vi "addCheckIN.vi"(0 "reference in":refnum<class "Project Panels.lvclass">=refnum, 11 "error in (no error)":errorcluster) -> (4 "reference out":refnum<class "Project Panels.lvclass">, 8 "saved?":bool, 15 "error out":errorcluster={"status"=TRUE, "code"=1556, "source"="In Place Element Structure in Project Panels.lvclass:addCheckIN.vi"})   [LabVIEW 2015, in "Project Panels.lvclass"]
uses:
  Project Panels.lvclass
  <vilib>/Utility/miscctls.llb/LVRowAndColumnTypeDef.ctl
  deviceState.ctl
  SYS/Items Controller_llb/Items Controller.lvclass
  APP/checkIN_class/checkIN.lvclass
panel:
  out "Cell Position":T1={"Row"=0, "Column"=4}
  out "title":string="Add Check IN"
  in  "getPDFFile":bool
  in  "updateData":bool
  in  "Quantity":i32
  in  "Description:":string
  in  "S/N:":string caption="Add more than one seprated by a \",\" without space"
  in  "P/N:":string
  out "dataIN":string[][](table)
  in  "Invoice Date:":string caption="(dd/mm/yyyy)"
  in  "Invoice Type:":string
  in  "Invoice Number:":string
  in  "ADD":bool
  in  "Date IN:":string caption="(dd/mm/yyyy)"
  out "Status bar":string="Fill in all and press the DONE button....."
  in  "Stop Button":bool
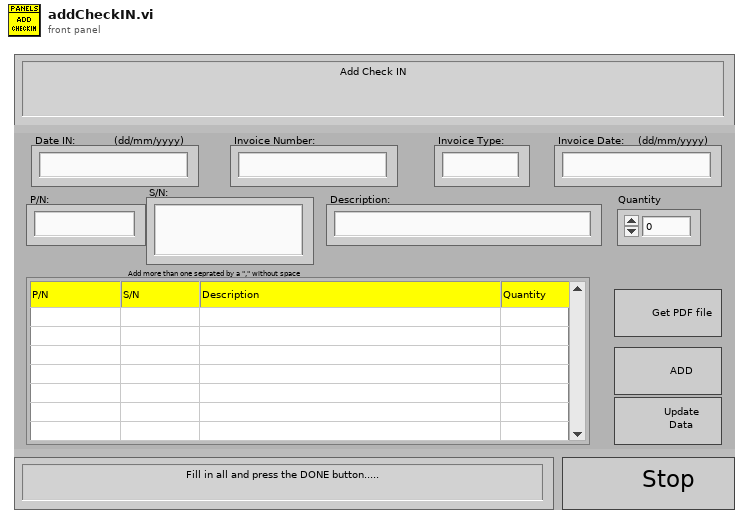
[diagram p1: front panel]
types:
  T1 = typedef "LVRowAndColumnTypeDef.ctl" = cluster{"Row":i32, "Column":i32}
  T2 = cluster{"P/N":string, "S/N":string, "Description":string, "Quantity":i32}
  T3 = typedef "Project Panels.lvclass/deviceState.ctl" = enum16{"check", "initiate", "waitEvent", "dataFromPDF", "getDetails", "TSR", "save", "close", "stop"}
  T4 = typedef "Project Panels.lvclass/ObjectAttributesRef.ctl" = refnum<data-value>
  T5 = typedef "Project Panels.lvclass/ObjectAttributes.ctl" = cluster{"MyAttribute":dbl, "device_controller_ref":refnum<class "Devices Controller.lvclass">, "file_controller_ref":refnum<class "File Controller.lvclass">, "item_controller_ref":refnum<class "Items Controller.lvclass">, "item_tables":cluster{"checkIN":string[][], "checkOUT":string[][], "storage":string[][]}, "quickbook_table":cluster{"notes":string[][]}, "notification_controller_ref":refnum<class "Notification Controller.lvclass">, "partstracking_controller_ref":refnum<class "PartsTracking Controller.lvclass">, "product_tables":cluster{"k4b2":string[][], "fitmate":string[][], "RMR":string[][], "CPET":string[][], "BP":string[][], "PP":string[][], "k5":string[][], "bb-pft":string[][]}, "rowsColour":u32[], "low_resolution?":bool}
  T6 = typedef "LVPoint32TypeDef.ctl" = cluster{"Horizontal":i32, "Vertical":i32}
  T7 = cluster{"checkIN_ref":refnum<class "checkIN.lvclass">, "checkOUT_ref":refnum<class "checkOUT.lvclass">, "item_ref":refnum<class "item.lvclass">}
  T8 = cluster{"numItems":string, "date":string, "numInvoice":string, "P/N":string[], "S/N":string[], "Descr":string[], "Qty":string[]}
  T9 = enum16{"Left Button", "Center Button", "Right Button", "Window Close"}
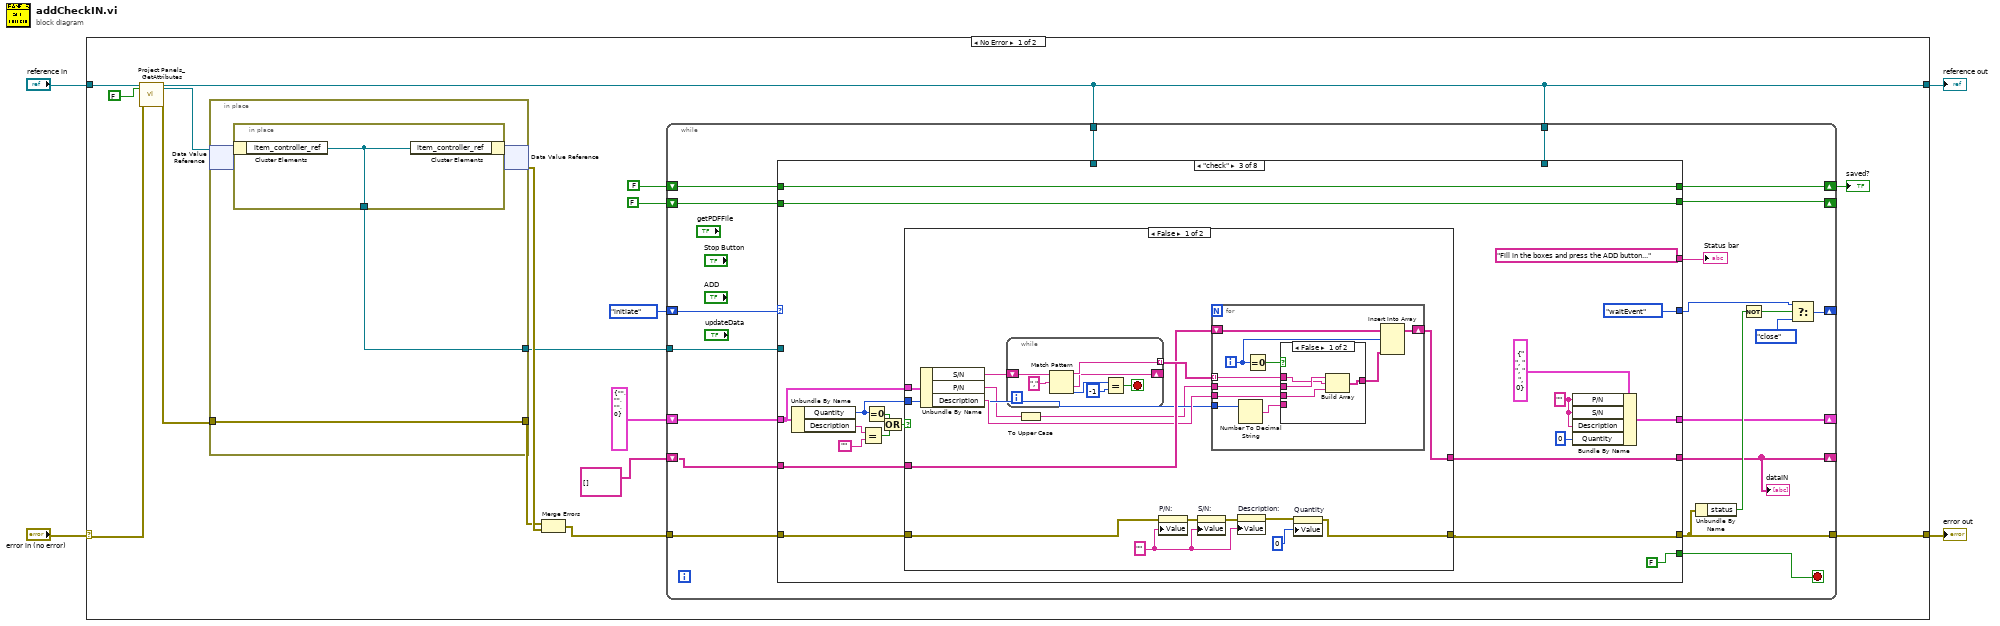
[diagram p0: block diagram]
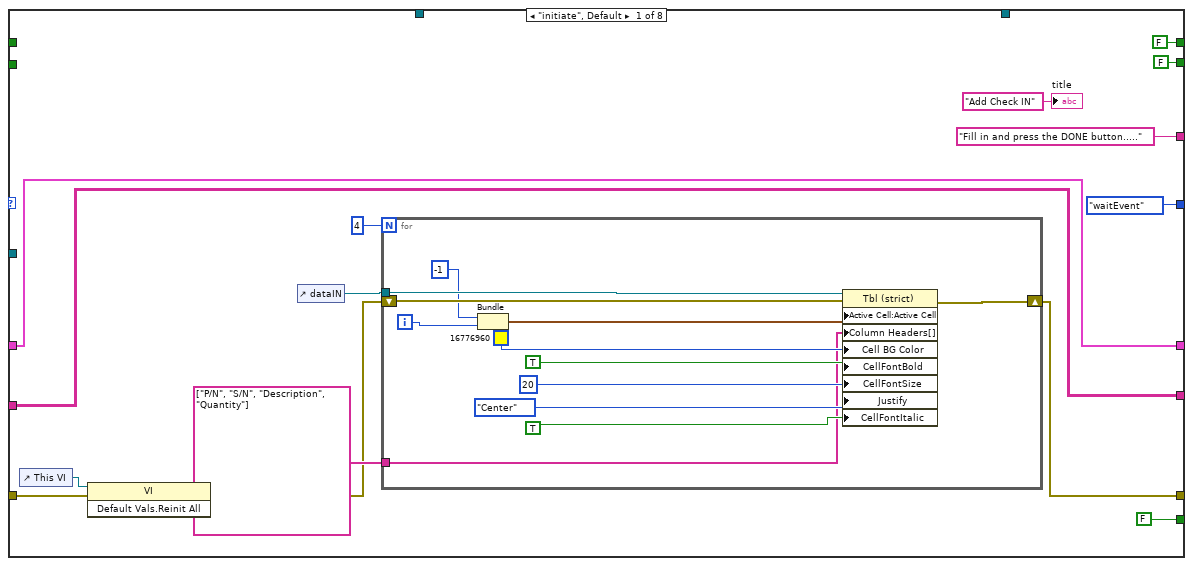
[diagram p2: hidden frame]
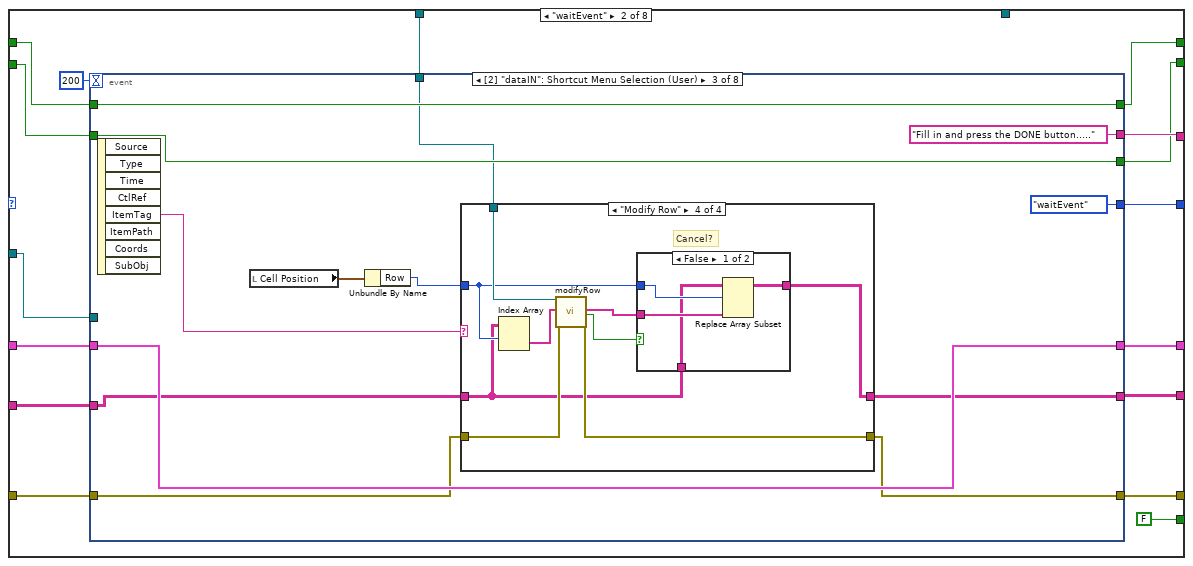
[diagram p3: hidden frame]
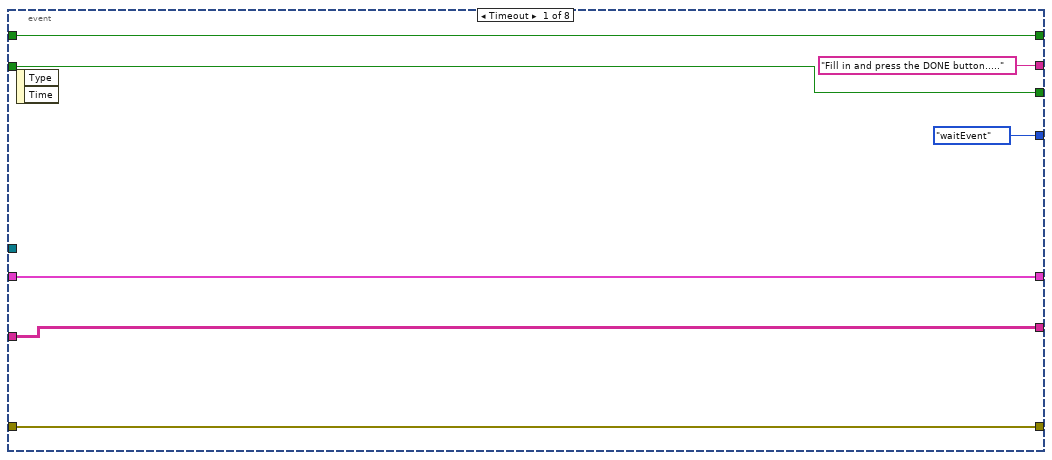
[diagram p4: hidden frame]
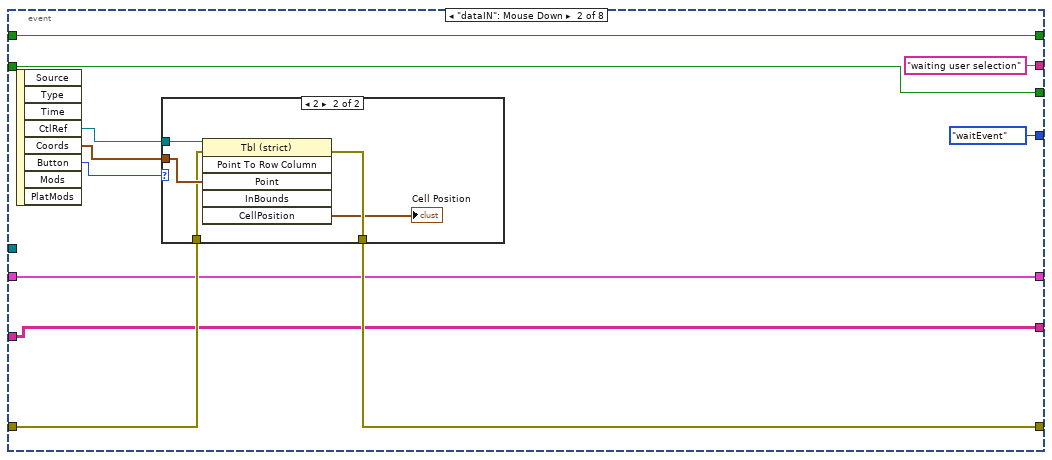
[diagram p5: hidden frame]
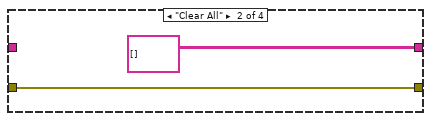
[diagram p8: hidden frame]
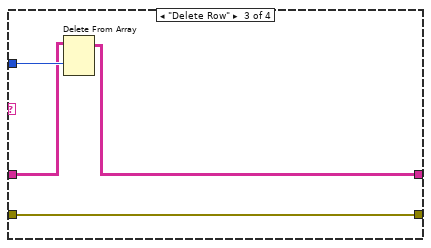
[diagram p9: hidden frame]
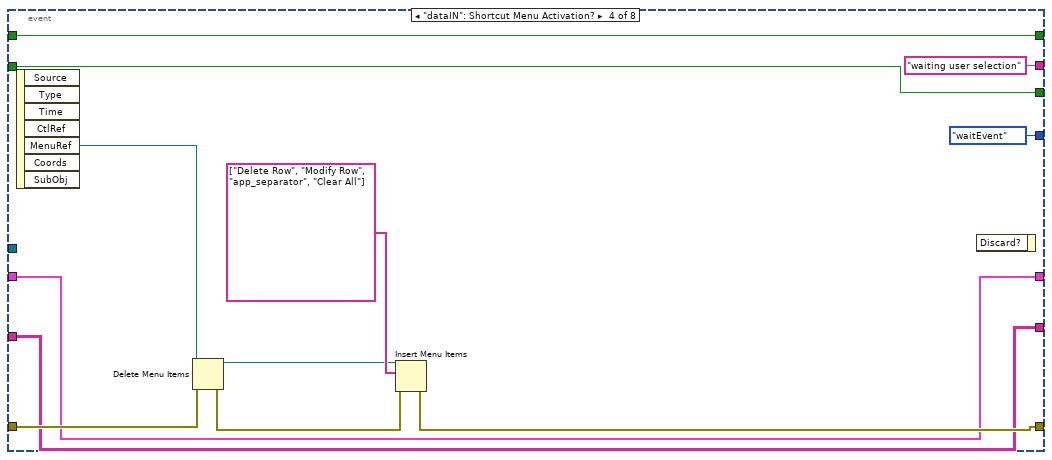
[diagram p11: hidden frame]
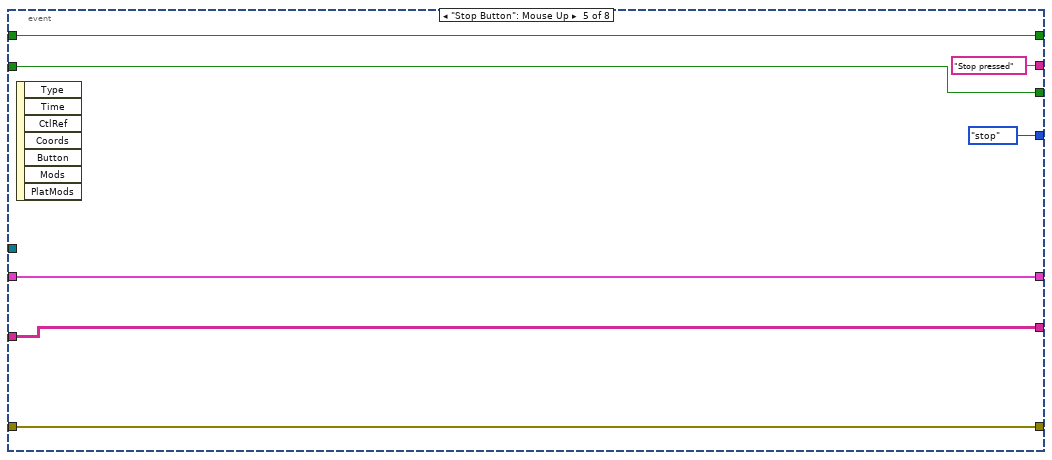
[diagram p12: hidden frame]
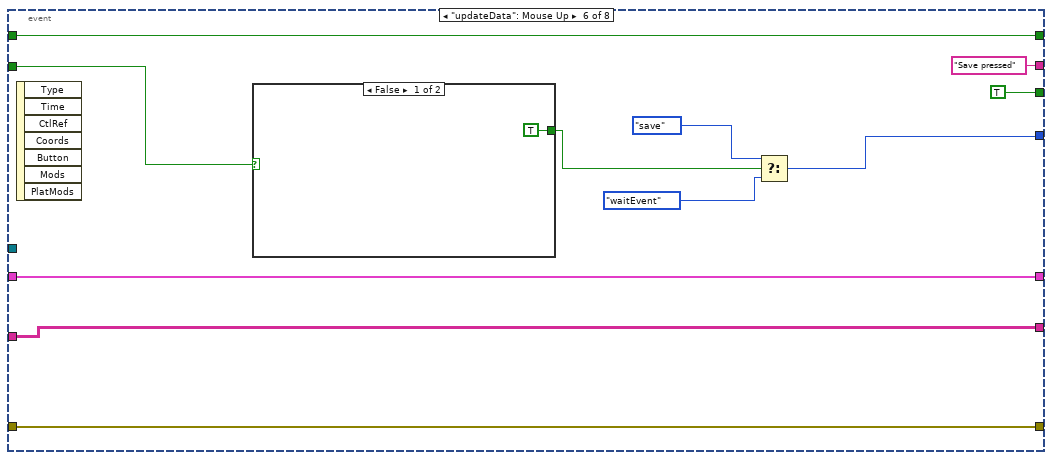
[diagram p13: hidden frame]
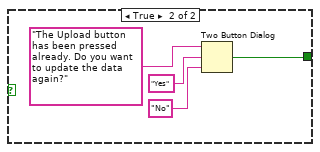
[diagram p14: hidden frame]
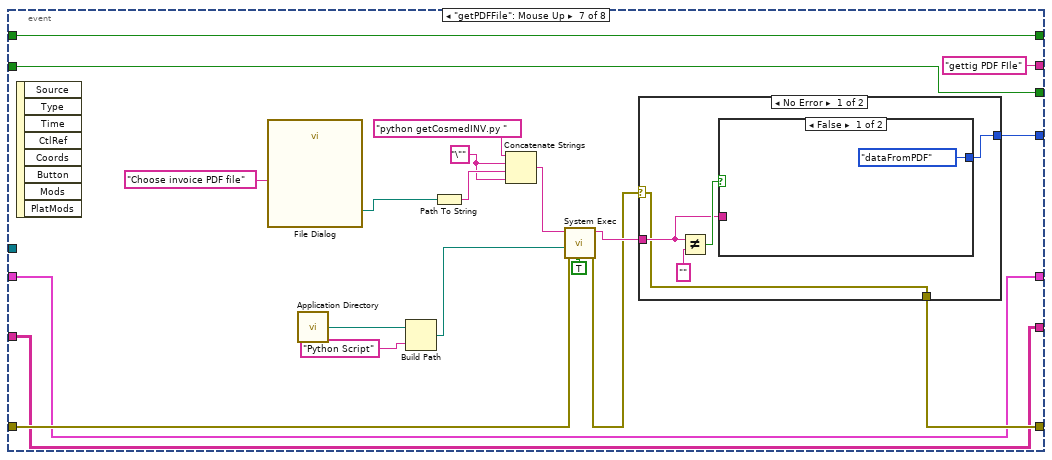
[diagram p15: hidden frame]
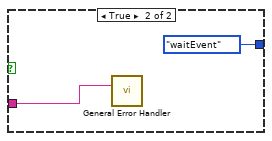
[diagram p16: hidden frame]
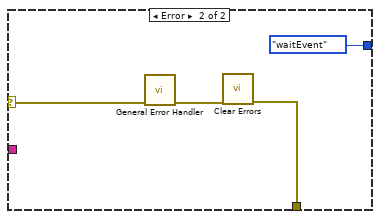
[diagram p17: hidden frame]
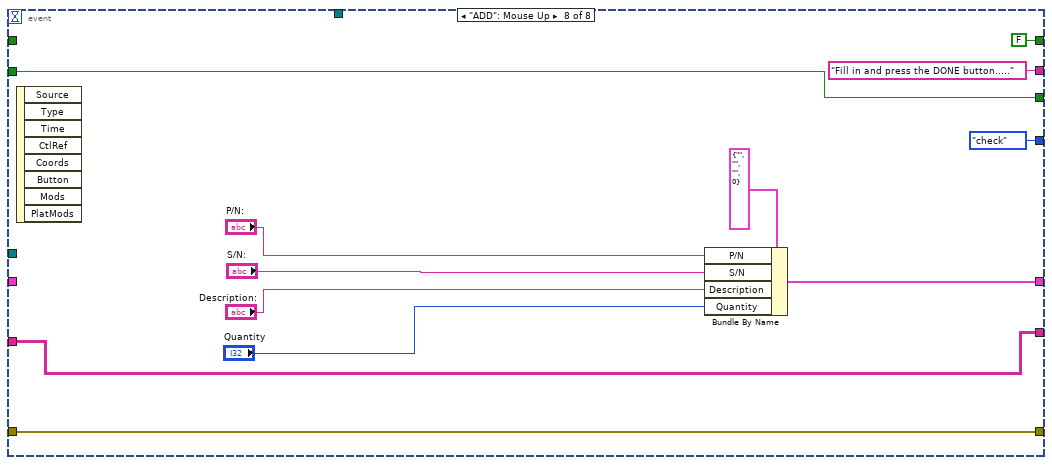
[diagram p18: hidden frame]
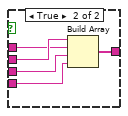
[diagram p19: hidden frame]
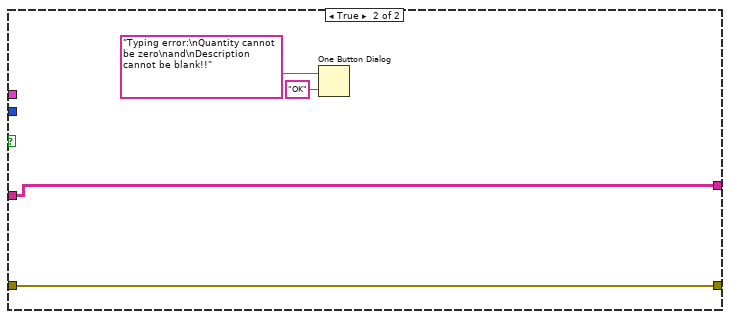
[diagram p20: hidden frame]
diagram:
  n1 = case shown="No Error" "error in (no error)" {
    selector: "error in (no error)" -> [w17 w422]
    tunnel: [w14 w422] -> w3
    tunnel: [w5 w421] -> w1
    tunnel: "reference in" -> [w19 w421]
    frame No Error {
      n2 = call "Project Panels_GetAttributes.vi"("reference in"=w19, "return data? (T)"=FALSE, "error in (no error)"=w17) -> ("reference out"=w5:refnum<class "Project Panels.lvclass">, "attributes ref"=w15:T4, "error out"=w16:errorcluster)  [unwired: 13 in, 1 out]
      n3 = in-place {
        in-place-border: w16 -> [w417]
        in-place-border: [w417] -> w20
        in-place-border: [w416] -> w11
        n4 = in-place-dvr #1(w15) -> (w418:T5)  [unwired: 1 out]
        n5 = in-place {
          in-place-border: [w420] -> w416
          n6 = in-place-cluster #2(w418) -> ("item_controller_ref"=w420:refnum<class "Items Controller.lvclass">)
          n7 = in-place-cluster #2("item_controller_ref"=w420) -> (w419:T5)
        }
        n8 = in-place-dvr #1(w419) -> (w21:errorcluster)  [unwired: 1 out]
      }
      n9 = Merge Errors(w20, w21) -> (w12:errorcluster)
      n10 = while {
        tunnel: w12 -> [w42]
        tunnel: [w24] -> w14
        shift-right: [w39] -> _
        shift-left: deviceState."initiate" ("state") -> [w41]
        tunnel: w5 -> [w35]
        tunnel: w11 -> [w33]
        shift-right: [w31] -> _
        shift-left: T2 {"P/N"="", "S/N"="", "Description"="", "Quantity"=0} -> [w30]
        shift-right: [w23] -> _
        shift-left: string[][] [] ("dataIN 2") -> [w29]
        shift-right: [w27] -> w7
        shift-left: FALSE -> [w28]
        shift-right: [w25] -> _
        shift-left: FALSE -> [w26]
        tunnel: w5 -> [w22]
        stop <- w34 stop-if-true
        n11 = case shown="\"check\"" w41 {
          tunnel: w42 -> [w53 w85 w240 w310 w335 w350 w381 w395]
          tunnel: [w48 w84 w231 w308 w335 w344 w381 w395] -> w24
          tunnel: [deviceState."waitEvent" ("state") w82 deviceState."waitEvent" ("f") deviceState."waitEvent" ("f") deviceState."stop" ("f") deviceState."waitEvent" ("f") deviceState."close" ("f") w391] -> w40
          tunnel: w35 -> [_ _ _ _ _ _ _ _]
          tunnel: [FALSE FALSE FALSE FALSE FALSE FALSE TRUE FALSE] -> w34
          tunnel: w33 -> [_ w73 _ w307 _ w351 _ _]
          tunnel: ["Fill in and press the DONE button....." ("Status bar") w80 "Fill in the boxes and press the ADD button..." ("Status bar") "Check data imported from PDF" ("Status bar") "" ("Status bar") "Wait while the new data are saved in the inventory" ("Status bar") "" ("Status bar") w392] -> w32
          tunnel: [w46 w79 w234 w306 w332 w356 w384 w394] -> w31
          tunnel: w30 -> [w46 w78 w236 w306 w332 w356 w384 w394]
          tunnel: w29 -> [w45 w77 w239 w299 w331 w341 w383 w393]
          tunnel: [w45 w76 w238 w298 w331 w341 w383 w393] -> w23
          tunnel: w28 -> [_ w75 w230 _ w330 _ w382 w390]
          tunnel: [FALSE w74 w230 FALSE w330 TRUE w382 w390] -> w27
          tunnel: w26 -> [_ w71 w224 w290 w329 w337 w380 w389]
          tunnel: [FALSE w72 w224 w290 w329 w337 w380 w389] -> w25
          tunnel: w22 -> [_ w70 _ _ _ _ _ _]
          frame "initiate", Default {
            n12 = control-ref of="This VI"() -> (w54:refnum<vi>)
            n13 = invoke class="VI" method="Default Vals.Reinit All"(reference=w54, error in=w53) -> (error out=w49:errorcluster)  [unwired: 1 in, 2 out]
            n14 = control-ref of="dataIN"() -> (w50:refnum<vi>)
            n15 = for {
              N: 4 -> [_]
              tunnel: w50 -> [w67]
              shift-right: [w68] -> w48
              shift-left: w49 -> [w69]
              tunnel: string[] ["P/N", "S/N", "Description", "Quantity"] ("Column Header Strings[]") -> [w58]
              i -> [w65]
              n16 = Bundle("index"=-1, w65) -> (w66:cluster{"index":i32, i32})  [unwired: 1 in]
              n17 = property on="Property Node" class="Tbl (strict)"(reference=w67, error in=w69, "Active Cell:Active Cell"=w66, "Column Headers[]"=w58, "Cell BG Color"=u32 16776960, "CellFontBold"=TRUE ("Active Cell:Cell Font:Bold"), "CellFontSize"=u32 20 ("Active Cell:Cell Font:Size"), "Justify"=enum16{"Left", "Center", "Right"}."Center" ("Active Cell:Cell Justification"), "CellFontItalic"=TRUE ("Active Cell:Cell Font:Italic")) -> (error out=w68:errorcluster)  [unwired: 1 out]
            }
            "title" <- "Add Check IN" ("title")
          }
          frame "waitEvent" {
            n18 = event shown="[2] \"dataIN\": Shortcut Menu Selection (User)" {
              selector: _ -> [_ _ _ _ _ _ _ _]
              dyn-events: _ -> [_ _ _ _ _ _ _ _]
              timeout: 200 -> [_ _ _ _ _ _ _ _]
              tunnel: w85 -> [w92 w103 w112 w154 w162 w174 w196 w223]
              tunnel: [w92 w102 w111 w152 w162 w174 w183 w223] -> w84
              tunnel: [deviceState."waitEvent" ("f") deviceState."waitEvent" ("f") deviceState."waitEvent" ("f") deviceState."waitEvent" ("f") deviceState."stop" ("f") w165 w186 deviceState."check" ("f")] -> w82
              tunnel: ["Fill in and press the DONE button....." ("Status bar") "waiting user selection" ("Status bar") "Fill in and press the DONE button....." ("Status bar") "waiting user selection" ("Status bar") "Stop pressed" ("Status bar") "Save pressed" ("Status bar") "gettig PDF FIle" ("Status bar") "Fill in and press the DONE button....." ("Status bar")] -> w80
              tunnel: [w89 w96 w122 w149 w160 w172 w181 w217] -> w79
              tunnel: w78 -> [w89 w96 w122 w149 w160 w172 w181 _]
              tunnel: w77 -> [w86 w97 w116 w150 w159 w171 w182 w214]
              tunnel: [w86 w97 w115 w150 w159 w171 w182 w214] -> w76
              tunnel: w75 -> [w88 w94 w119 w145 w158 w170 w198 _]
              tunnel: [w88 w94 w119 w145 w158 w170 w198 FALSE] -> w74
              tunnel: w73 -> [_ _ _ _ _ _ _ _]
              tunnel: [w87 w95 w120 w146 w157 TRUE w180 w212] -> w72
              tunnel: w71 -> [w87 w95 w120 w146 w157 w168 w180 w212]
              tunnel: w70 -> [_ _ w110 _ _ _ _ _]
              event Timeout {
                n19 = event-data() -> ()  [unwired: 1 in, 2 out]
              }
              event "dataIN": Mouse Down {
                n20 = event-data() -> ("CtlRef"=w99:refnum<vi>, "Coords"=w100:T6, "Button"=w101:u16)  [unwired: 1 in, 5 out]
                n21 = case shown="2" w101 {
                  tunnel: w99 -> [_ w109]
                  tunnel: w100 -> [_ w108]
                  tunnel: w103 -> [w104 w107]
                  tunnel: [w104 w106] -> w102
                  frame 0, Default {
                  }
                  frame 2 {
                    n22 = invoke class="Tbl (strict)" method="Point To Row Column"(reference=w109, error in=w107, "Point"=w108) -> (error out=w106:errorcluster, "CellPosition"=→"Cell Position":T1)  [unwired: 3 in, 4 out]
                  }
                }
              }
              event "dataIN": Shortcut Menu Selection (User) {
                n23 = event-data() -> ("ItemTag"=w114:string)  [unwired: 1 in, 7 out]
                n24 = local read "Cell Position"() -> (w117:T1)
                n25 = Unbundle By Name(w117) -> ("Row"=w113:i32)
                n26 = case shown="\"Modify Row\"" w114 {
                  tunnel: w116 -> [w124 _ w129 w133]
                  tunnel: [w124 string[][] [] ("dataIN 2") w128 w137] -> w115
                  tunnel: w113 -> [_ _ w130 w134]
                  tunnel: w112 -> [w123 w125 w127 w139]
                  tunnel: [w123 w125 w127 w138] -> w111
                  tunnel: w110 -> [_ _ _ w135]
                  frame "False", Default {
                  }
                  frame "Clear All" {
                  }
                  frame "Delete Row" {
                    n27 = Delete From Array(array=w129, index (row)=w130) -> (array with subset deleted=w128:string[][])  [unwired: 2 in, 1 out]
                  }
                  frame "Modify Row" {
                    # "Cancel?"
                    n28 = Index Array(array=w133, index (row)=w134) -> (element=w132:string[])  [unwired: 1 in]
                    n29 = call-dynamic "modifyRow.vi"("reference in"=w135, "Row In"=w132, "error in (no error)"=w139) -> ("Row"=w136:string[], "Cancel?"=w131:bool, "error out"=w138:errorcluster)  [unwired: 13 in, 1 out]
                    n30 = case shown="False" w131 {
                      tunnel: [w143 w144] -> w137
                      tunnel: w136 -> [w142 _]
                      tunnel: w134 -> [w141 _]
                      tunnel: w133 -> [w140 w144]
                      frame False {
                        n31 = Replace Array Subset(array=w140, new element=w142, index (row)=w141) -> (w143:string[][])  [unwired: 1 in]
                      }
                      frame True {
                      }
                    }
                  }
                }
              }
              event "dataIN": Shortcut Menu Activation? {
                n32 = event-data() -> ("MenuRef"=w151:refnum<k9>)  [unwired: 1 in, 6 out]
                n33 = Delete Menu Items(6:w154, 9:w151) -> (0:w153:errorcluster, 3:w155:refnum<k9>)  [unwired: 2 in]
                n34 = Insert Menu Items(6:w153, 8:string[] ["Delete Row", "Modify Row", "app_separator", "Clear All"] ("item names"), 9:w155) -> (0:w152:errorcluster)  [unwired: 3 in, 2 out]
                n35 = event-data() -> ()  [unwired: 2 in, 1 out]
              }
              event "Stop Button": Mouse Up {
                n36 = event-data() -> ()  [unwired: 1 in, 7 out]
              }
              event "updateData": Mouse Up {
                n37 = event-data() -> ()  [unwired: 1 in, 7 out]
                n38 = case shown="False" w168 {
                  tunnel: [TRUE ("T button?") w176] -> w167
                  frame False {
                  }
                  frame True {
                    n39 = Two Button Dialog(message="The Upload button has been pressed already. Do you want to update the data again?", 1:"No" ("F button name (\"Cancel\")"), 2:"Yes" ("T button name (\"OK\")")) -> (T button?=w176:bool)
                  }
                }
                n40 = Select(t=deviceState."save" ("f"), s=w167, f=deviceState."waitEvent") -> (s? t:f=w165:T3)
              }
              event "getPDFFile": Mouse Up {
                w191 = "\"" ("string")
                n41 = event-data() -> ()  [unwired: 1 in, 8 out]
                n42 = call "File Dialog"("prompt"="Choose invoice PDF file") -> ("selected path"=w195:path)  [unwired: 11 in, 3 out]
                n43 = call <vilib>:"Application Directory.vi"() -> ("Application Directory"=w189:path)
                n44 = Build Path(base path=w189, name or relative path="Python Script" ("string")) -> (appended path=w187:path)
                n45 = Path To String(path=w195) -> (string=w192:string)
                n46 = Concatenate Strings("python getCosmedINV.py " ("command line"), w191, w192, w191) -> (w190:string)
                n47 = call <vilib>:"System Exec.vi"("run minimized? (F)"=TRUE, "error in (no error)"=w196, "working directory"=w187, "command line"=w190) -> ("error out"=w184:errorcluster, "standard output"=w185:string)  [unwired: 2 in, 4 out]
                n48 = case shown="No Error" w184 {
                  selector: w184 -> [w200 w210]
                  tunnel: [w202 deviceState."waitEvent" ("f")] -> w186
                  tunnel: w185 -> [w201 _]
                  tunnel: [w200 w208] -> w183
                  frame No Error {
                    n49 = Not Equal?(x=w201, y="") -> (x != y?=w203:bool)
                    n50 = case shown="False" w203 {
                      tunnel: w201 -> [_ w206]
                      tunnel: [deviceState."dataFromPDF" ("f") deviceState."waitEvent" ("f")] -> w202
                      frame False {
                      }
                      frame True {
                        n51 = call <vilib>:"General Error Handler.vi"("[error source] (\" \")"=w206) -> ()  [unwired: 10 in, 5 out]
                      }
                    }
                  }
                  frame Error {
                    n52 = call <vilib>:"General Error Handler.vi"("error in (no error)"=w210) -> ("error out"=w209:errorcluster)  [unwired: 10 in, 4 out]
                    n53 = call <vilib>:"Clear Errors.vi"("error in (no error)"=w209) -> ("error out"=w208:errorcluster)  [unwired: 5 in, 1 out]
                  }
                }
              }
              event "ADD": Mouse Up {
                n54 = event-data() -> ()  [unwired: 1 in, 8 out]
                n55 = Bundle By Name(cluster=T2 {"P/N"="", "S/N"="", "Description"="", "Quantity"=0}, "P/N"="P/N:", "S/N"="S/N:", "Description"="Description:", "Quantity"="Quantity") -> (w217:T2)
              }
            }
          }
          frame "check" {
            w233 = "" ("P/N")
            n56 = Unbundle By Name(w236) -> ("Quantity"=w237:i32, "Description"=w229:string)
            n57 = Equal?(x=w229, y="") -> (x = y?=w226:bool)
            n58 = Equal To 0?(x=w237) -> (x = 0?=w225:bool)
            n59 = Or(x=w225, y=w226) -> (x .or. y?=w227:bool)
            n60 = case shown="False" w227 {
              tunnel: w240 -> [w247 w289]
              tunnel: [w246 w289] -> w231
              tunnel: w239 -> [w257 w286]
              tunnel: [w253 w286] -> w238
              tunnel: w237 -> [w254 _]
              tunnel: w236 -> [w259 _]
              frame False {
                w251 = "" ("P/N:")
                n61 = Unbundle By Name(w259) -> ("S/N"=w256:string, "P/N"=w245:string, "Description"=w255:string)
                n62 = while {
                  tunnel: [w284] -> w258 mode=indexing
                  shift-right: [w280] -> _
                  shift-left: w256 -> [w279]
                  stop <- w283 stop-if-true
                  n63 = Match Pattern(string=w279, regular expression=",") -> (before substring=w284:string, after substring=w280:string, offset past match=w282:i32)  [unwired: 1 in, 1 out]
                  n64 = Equal?(x=w282, y=-1) -> (x = y?=w283:bool)
                }
                n65 = To Upper Case(1:w245) -> (0:w244:string)
                n66 = property on="P/N:" class="Str"(error in=w247, "Value"=w251) -> (error out=w248:errorcluster)  [unwired: 1 in, 1 out]
                n67 = property on="S/N:" class="Str"(error in=w248, "Value"=w251) -> (error out=w249:errorcluster)  [unwired: 1 in, 1 out]
                n68 = for {
                  tunnel: w258 -> [w268] mode=indexing
                  tunnel: w244 -> [w269]
                  tunnel: w255 -> [w267]
                  shift-right: [w265] -> w253
                  shift-left: w257 -> [w266]
                  tunnel: w254 -> [w263]
                  i -> [w260]
                  n69 = Number To Decimal String(number=w263) -> (decimal integer string=w262:string)  [unwired: 1 in]
                  n70 = Equal To 0?(x=w260) -> (x = 0?=w261:bool)
                  n71 = case shown="False" w261 {
                    tunnel: w269 -> [w271 w278]
                    tunnel: w268 -> [w270 w277]
                    tunnel: w267 -> [w272 w276]
                    tunnel: [w273 w275] -> w264
                    tunnel: w262 -> [_ w274]
                    frame False {
                      n72 = Build Array(w271, w270, w272) -> (w273:string[])
                    }
                    frame True {
                      n73 = Build Array(w278, w277, w276, w274) -> (w275:string[])
                    }
                  }
                  n74 = Insert Into Array(array=w266, index (row)=w260, new element=w264) -> (w265:string[][])  [unwired: 1 in]
                }
                n75 = property on="Description:" class="Str"(error in=w249, "Value"=w251) -> (error out=w250:errorcluster)  [unwired: 1 in, 1 out]
                n76 = property on="Quantity" class="DigNum (strict)"(error in=w250, "Value"=0 ("Quantity")) -> (error out=w246:errorcluster)  [unwired: 1 in, 1 out]
              }
              frame True {
                n77 = One Button Dialog(message="Typing error:\nQuantity cannot be zero\nand\nDescription cannot be blank!!", button name ("OK")="OK") -> ()  [unwired: 1 out]
              }
            }
            n78 = Bundle By Name(cluster=T2 {"P/N"=" ", "S/N"=" ", "Description"=" ", "Quantity"=0}, "P/N"=w233, "S/N"=w233, "Description"=w233, "Quantity"=0) -> (w234:T2)
          }
          frame "dataFromPDF" {
            n79 = call "getItemsRefs.vi"("error in (no error)"=w310, "reference in"=w307) -> ("error out"=w309:errorcluster, "itemsRef"=w312:T7)  [unwired: 7 in, 1 out]
            n80 = call <vilib>:"Application Directory.vi"() -> ("Application Directory"=w305:path)
            n81 = Unbundle By Name(w312) -> ("checkIN_ref"=w311:refnum<class "checkIN.lvclass">)
            n82 = Get Date/Time In Seconds() -> (seconds since 1Jan1904=w291:timestamp)
            n83 = Build Path(base path=w305, name or relative path="Python Script\\results.txt" ("string")) -> (appended path=w303:path)
            n84 = Get Date/Time String(seconds (now)=w291) -> (date string=w292:string)  [unwired: 2 in, 1 out]
            n85 = call "getPDFData.vi"("reference in"=w311, "file (use dialog)"=w303, "error in (no error)"=w309) -> ("dataOUT"=w302:T8, "error out"=w308:errorcluster)  [unwired: 14 in, 1 out]
            n86 = Unbundle By Name(w302) -> ("date"=w300:string, "numInvoice"=w301:string, "P/N"=w297:string[], "S/N"=w296:string[], "Descr"=w295:string[], "Qty"=w294:string[])
            n87 = local write "Invoice Type:"("REM" ("Invoice Type:")) -> ()
            n88 = local write "Date IN:"(w292) -> ()
            n89 = local write "Invoice Number:"(w301) -> ()
            n90 = local write "Invoice Date:"(w300) -> ()
            n91 = for {
              tunnel: w297 -> [w323] mode=indexing
              tunnel: w296 -> [w318] mode=indexing
              tunnel: w295 -> [w322] mode=indexing
              shift-right: [w325] -> w298
              shift-left: w299 -> [w326]
              tunnel: w294 -> [w321] mode=indexing
              n92 = Equal?(x=w318, y="none") -> (x = y?=w319:bool)
              n93 = case shown="True" w319 {
                tunnel: w318 -> [w327 _]
                tunnel: [w327 ""] -> w317
                frame False {
                }
                frame True {
                }
              }
              n94 = Build Array(w323, w317, w322, w321) -> (w324:string[])
              n95 = Insert Into Array(array=w326, new element=w324) -> (w325:string[][])  [unwired: 2 in]
            }
          }
          frame "getDetails" {
          }
          frame "save" {
            n96 = for {
              tunnel: w341 -> [w374] mode=indexing
              tunnel: "Date IN:" -> [w379]
              tunnel: "Invoice Number:" -> [w378]
              tunnel: "Invoice Type:" -> [w377]
              tunnel: "Invoice Date:" -> [w376]
              tunnel: [w375] -> w347 mode=indexing
              n97 = Build Array (concatenate)(w379, w374, w378, w377, w376) -> (w375:string[])
            }
            n98 = call "updateIN-OUT.vi"("error in (no error)"=w350, "IN-OUT"=FALSE, "dataIN"=w347, "reference in"=w351) -> ("error out"=w345:errorcluster, "reference out"=w348:refnum<class "Items Controller.lvclass">)  [unwired: 6 in]
            n99 = for {
              tunnel: [w363] -> w340 mode=indexing
              tunnel: w341 -> [w361] mode=indexing
              w362 = "storage"
              # "add position,\nlocation and\nnotes"
              n100 = Build Array (concatenate)(w361, w362, w362, "" ("element")) -> (w363:string[])
            }
            n101 = call "updateStorage.vi"("error in (no error)"=w345, "IN-OUT"=FALSE, "dataIN"=w340, "reference in"=w348) -> ("error out"=w344:errorcluster, "warningMess"=w339:string[])  [unwired: 5 in, 1 out]
            n102 = Array Size(array=w339) -> (size(s)=w343:i32)
            n103 = Equal To 0?(x=w343) -> (x = 0?=w342:bool)
            n104 = case shown="False" w342 {
              tunnel: w339 -> [w369 _]
              frame False {
                n105 = for {
                  tunnel: w369 -> [w371] mode=indexing
                  shift-right: [w373] -> w367
                  shift-left: "" -> [w372]
                  n106 = Concatenate Strings(w372, w371, "\r\n") -> (w373:string)
                }
                n107 = Concatenate Strings("The P/N is not cosmed or\nS/N already present for the following items:\n", w367, "Please update the storage for the missing P/N.") -> (w365:string)
                n108 = One Button Dialog(message=w365) -> ()  [unwired: 1 in, 1 out]
              }
              frame True {
              }
            }
          }
          frame "close" {
            n109 = case shown="Error" w381 {
              selector: w381 -> [_ w388]
              frame No Error {
              }
              frame Error {
                n110 = call <vilib>:"General Error Handler.vi"("error in (no error)"=w388) -> ()  [unwired: 10 in, 5 out]
              }
            }
          }
          frame "stop" {
            n111 = Unbundle By Name(w395) -> ("status"=w396:bool)
            n112 = case shown="False" w396 {
              tunnel: w395 -> [_ w413]
              tunnel: ["Stop pressed" w412] -> w392
              tunnel: [w399 deviceState."close" ("f")] -> w391
              tunnel: w390 -> [w398 _]
              frame False {
                n113 = case shown="False" w398 {
                  tunnel: [w401 deviceState."close" ("f")] -> w399
                  frame False {
                    n114 = call <vilib>:"Three Button Dialog.vi"("Window Title (\"\")"="Warning message" ("Window Title (\"\")"), "Right Button Text (\"Cancel\")"="Save" ("Right Button Text (\"Cancel\")"), "message"="You are closing the panel withoug updating the data.\nDo you wanna close it anyway?") -> ("Which Button?"=w402:T9)  [unwired: 8 in]
                    n115 = case shown="\"Left Button\", Default" w402 {
                      tunnel: [deviceState."close" ("f") deviceState."waitEvent" ("f") deviceState."save" ("f") deviceState."waitEvent" ("f")] -> w401
                      frame "Left Button", Default {
                      }
                      frame "Center Button" {
                      }
                      frame "Right Button" {
                      }
                      frame "Window Close" {
                      }
                    }
                  }
                  frame True {
                  }
                }
              }
              frame True {
                n116 = Unbundle By Name(w413) -> ("source"=w414:string)
                n117 = Concatenate Strings("An error occur: " ("message"), w414) -> (w412:string)
                n118 = One Button Dialog(message=w412) -> ()  [unwired: 1 in, 1 out]
              }
            }
          }
        }
        "dataIN" <- w23
        "Status bar" <- w32
        n119 = Unbundle By Name(w24) -> ("status"=w38:bool)
        n120 = Not(x=w38) -> (.not. x?=w37:bool)
        n121 = Select(t=w40, s=w37, f=deviceState."close") -> (s? t:f=w39:T3)
      }
      "saved?" <- w7
    }
    frame Error {
    }
  }
  "error out" <- w3
  "reference out" <- w1
